vi "Download.vi"(8 "error in":errorcluster, 9 "Timeout":i32=1000 format="%d ms", 10 "Parameters":T4 {"Data" format="%02x"; "Multiplexer"."Sub Index" format="%02x"; "Multiplexer"."Index" format="%04x"}, 11 "SDO Manager in":refnum<class "SDO Manager.lvclass">) -> (0 "error out":errorcluster, 2 "SDO Result":T1={"Success"=FALSE, "SDO abort code"={"Null"=TRUE, "Value"=84082688}, "Data"={"Null"=TRUE, "Data"=[]}} {"SDO abort code"."Value" items=["Toggle bit not allowed"=84082688, "SDO protocol timed out"=84148224, "Client/server command specifier not valid or unknown"=84148225, "Invalid block size (block mode only)"=84148226, "Invalid sequence number (block mode only)"=84148227, "CRC error (block mode only)"=84148228, "Out of memory"=84148229, "Attempt to read a write only object"=100728833, "Attempt to write a read only object"=100728834, "Object does not exist in the object dictionary"=100794368, "Object cannot be mapped to the PDO"=100925505, "The number and length of the objects to be mapped would exceed PDO length"=100925506, "General parameter incompatibility reason"=100925507, "General internal incompatibility in the device"=100925511, "Access failed due to an hardware error"=101056512, "Data type does not match, length of service parameter does not match"=101122064, "Data type does not match, length of service parameter too high"=101122066, "Data type does not match, length of service parameter too low"=101122067, "Sub-index does not exist"=101253137, "Invalid value for parameter (download only)"=101253168, "Value of parameter written too high (download only)"=101253169, "Value of parameter written too low (download only)"=101253170, "Maximum value is less than minimum value"=101253174, "Resource not available: SDO connection"=101318691, "General error"=134217728, "Data cannot be transferred or stored to the application"=134217760, "Data cannot be transferred or stored to the application because of local control"=134217761, "Data cannot be transferred or stored to the application because of the present device stable"=134217762, "Object dictionary dynamic generation fails or no object dictionary is present (e.g. object dictionary is generated from file and generation fails because of an file error)"=134217763, "No data available"=134217764]; "Data"."Data" format="%02x"}, 3 "SDO Manager out":refnum<class "SDO Manager.lvclass">)   [LabVIEW 2020, in "CANopen.lvlib" / "SDO Manager.lvlib" / "SDO Manager.lvclass"]
uses:
  SDO Manager.lvclass
  Expedited Download Transfer/Expedited Download Transfer.lvclass
  SDO Manager.lvclass/SDO Manager.ctl
  Typedefs/SDO Result.ctl
  SDO Transfer/SDO Transfer.lvclass
  Typedefs/Multiplexer.ctl
  CANopen.lvlib
  SDO Transfer/SDO abort code.ctl
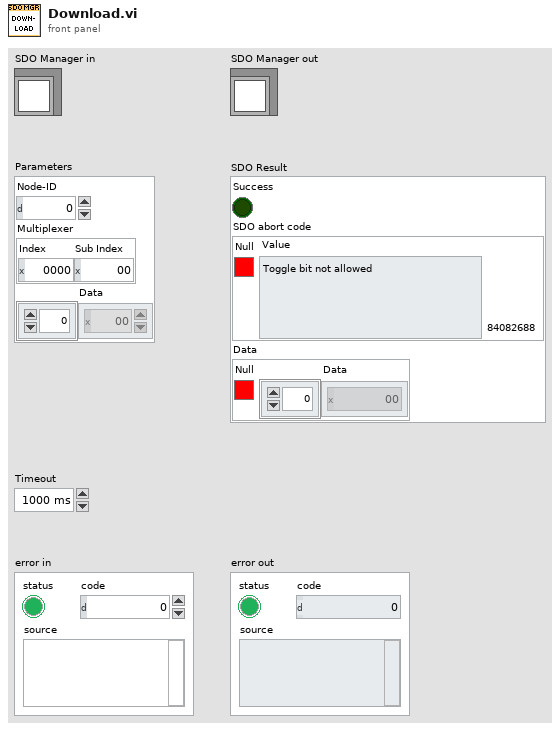
[diagram p1: front panel]
types:
  T1 = typedef "CANopen.lvlib/SDO Manager.lvlib/SDO Transfer.lvclass/SDO Result.ctl" = cluster{"Success":bool, "SDO abort code":cluster{"Null":bool, "Value":T2}, "Data":cluster{"Null":bool, "Data":u8[]}}
  T2 = typedef "CANopen.lvlib/SDO Manager.lvlib/SDO Transfer.lvclass/SDO abort code.ctl" = u32
  T3 = typedef "CANopen.lvlib/Multiplexer.ctl" = cluster{"Index":u16, "Sub Index":u8}
  T4 = cluster{"Node-ID":u8, "Multiplexer":T3, "Data":u8[]}
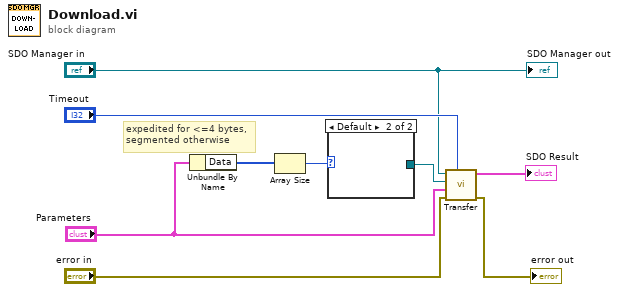
[diagram p0: block diagram]
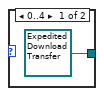
[diagram p2: hidden frame]
diagram:
  # "expedited for <=4 bytes,\nsegmented otherwise"
  n1 = Unbundle By Name("Parameters") -> ("Data"=w9:u8[])
  n2 = Array Size(array=w9) -> (size(s)=w7:i32)
  n3 = case shown="Default" w7 {
    tunnel: [refnum<class "Expedited Download Transfer.lvclass"> refnum ("CANopen Master:Expedited Transfer.lvclass") _] -> w5
    frame 0..4 {
    }
    frame Default {
    }
  }
  n4 = call "Transfer.vi"("Retry Delay"="Timeout", "error in"="error in", "Parameters"="Parameters", "SDO Transfer"=w5, "SDO Manager in"="SDO Manager in") -> ("error out"=→"error out":errorcluster, "SDO Result"=→"SDO Result":T1)  [unwired: 5 in]
  "SDO Manager out" <- "SDO Manager in"
